vi "Acquire Color Image with Skeletal Mapping.vi"() -> ()   [LabVIEW 2014]
uses:
  support/kinectRead [DepthFrame].vi
  support/kinectRead [BodyFrame].vi
panel:
  out "Body Index Image":T1(plugin-control)
  in  "stop":bool
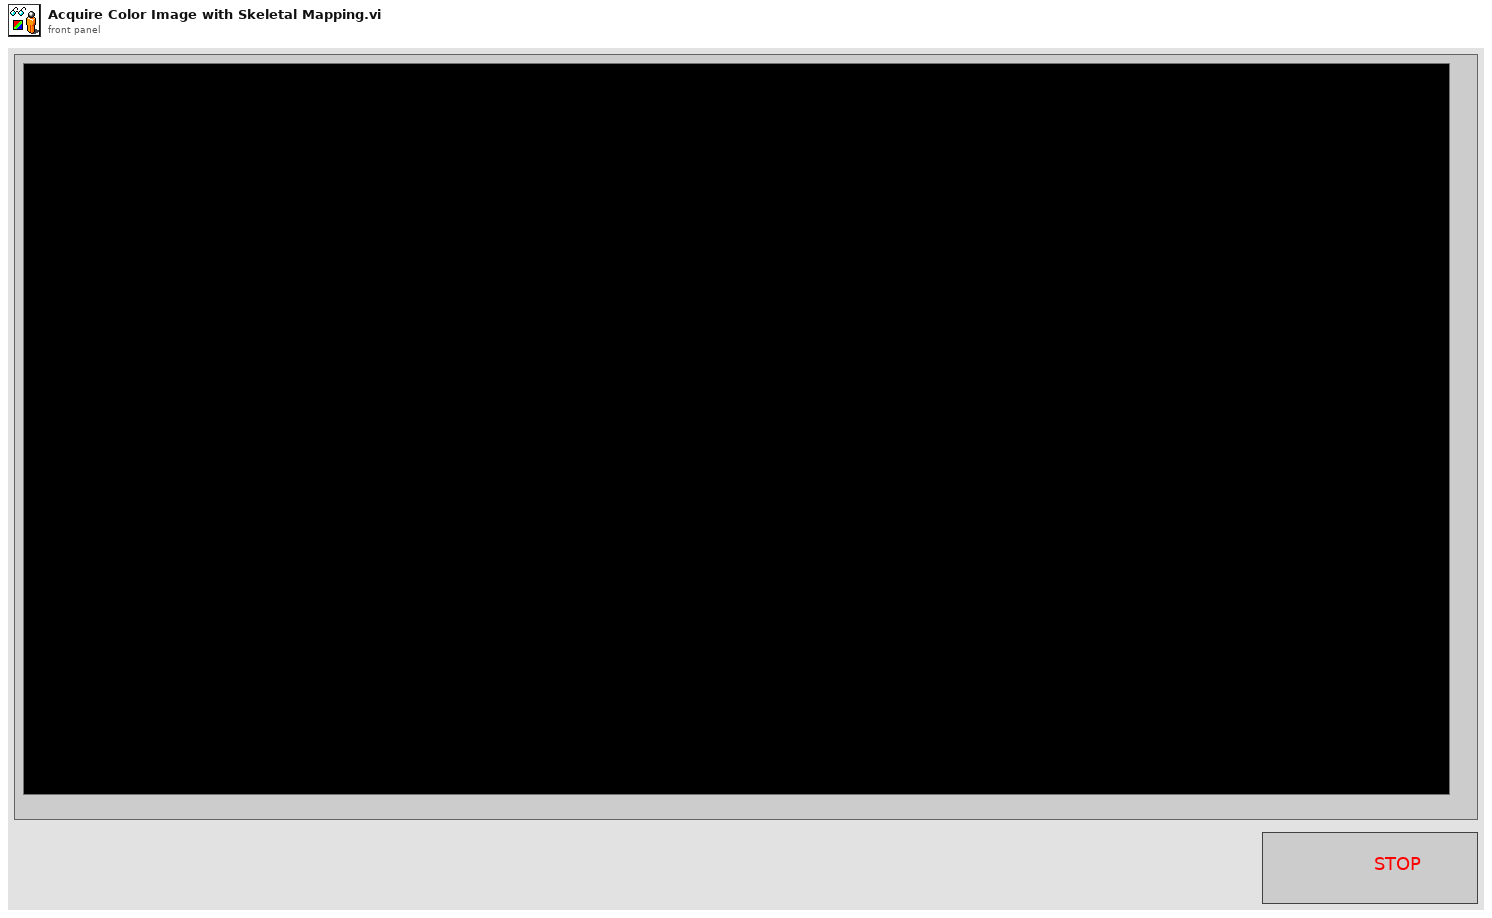
[diagram p1: front panel]
types:
  T1 = typedef "IMAQ Image.ctl" = refnum<image>
  T2 = typedef "Image Type" = u32
  T3 = typedef "KinectSensor References.ctl" = cluster{"KinectSensor":refnum<k24>, "MultiSourceFrameReader":refnum<k24>, "BodyFrameDataInterface":refnum<k24>}
  T4 = typedef "BodyData.ctl" = cluster{"ClippedEdges":i32, "HandLeftConfidence":i32, "HandLeftState":i32, "HandRightConfidence":i32, "HandRightState":i32, "IsRestricted":bool, "IsTracked":bool, "JointOrientations":refnum<k24>, "Joints":refnum<k24>, "Lean":refnum<k24>, "LeanTrackingState":i32, "TrackingId":u64}
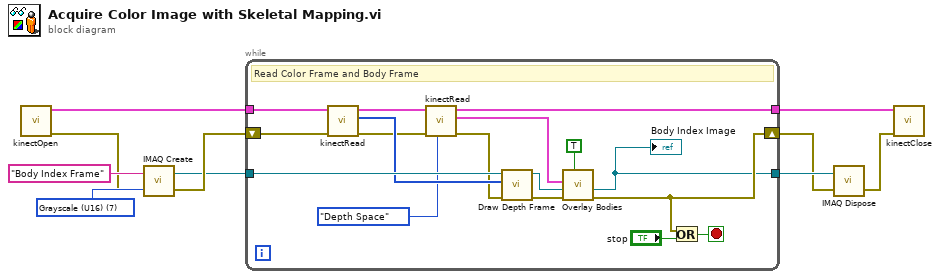
[diagram p0: block diagram]
diagram:
  w10 = T2 7 items=["Grayscale (U8)", "Grayscale (I16)", "Grayscale (SGL)", "Complex (CSG)", "RGB (U32)", "HSL (U32)", "RGB (U64)", "Grayscale (U16)"] ("Image Type")
  n1 = call "kinectOpen.vi"() -> ("error out"=w1:errorcluster, "KinectSensor References out"=w2:T3)  [unwired: 10 in]
  n2 = call "IMAQ Create"("Image Name"="Body Index Frame", "Image Type"=w10, "error in (no error)"=w1) -> ("New Image"=w8:T1, "error out"=w9:errorcluster)  [unwired: 2 in]
  n3 = while {
    tunnel: w2 -> [w27]
    shift-right: [w15] -> w6
    shift-left: w9 -> [w26]
    tunnel: w8 -> [w23]
    tunnel: [w14] -> w7
    tunnel: [w12] -> w3
    stop <- w24 stop-if-true
    # "Read Color Frame and Body Frame"
    n4 = call-poly "kinectRead.vi"("error in (no error)"=w26, "KinectSensor References in"=w27) -> ("error out"=w21:errorcluster, "frameData"=w22:u16[], "KinectSensor References out"=w20:T3)  [unwired: 7 in]
    n5 = call-poly "kinectRead.vi"("Coordinate Space"=enum16{"Color Space", "Depth Space"}."Depth Space", "error in (no error)"=w21, "KinectSensor References in"=w20) -> ("error out"=w19:errorcluster, "Body Data"=w16:T4[], "KinectSensor References out"=w12:T3)  [unwired: 6 in]
    n6 = call "Draw Depth Frame.vi"("error in (no error)"=w19, "U16 Array"=w22, "Image"=w23) -> ("error out"=w17:errorcluster, "Image Out"=w18:T1)  [unwired: 7 in]
    n7 = call "Overlay Bodies.vi"("Include Inferred Joints?"=TRUE, "error in"=w17, "Image"=w18, "Body Data"=w16) -> ("error out"=w15:errorcluster, "Image Out"=w14:T1)  [unwired: 6 in]
    "Body Index Image" <- w14
    n8 = Or(x=w15, y="stop") -> (x .or. y?=w24:bool)
  }
  n9 = call "IMAQ Dispose"("Image"=w7, "error in (no error)"=w6) -> ("error out"=w5:errorcluster)  [unwired: 4 in]
  n10 = call "kinectClose.vi"("error in"=w5, "KinectSensor References"=w3) -> ()  [unwired: 9 in, 1 out]
